vi "Register for Camera Events.vi"(8 "error in (no error)":errorcluster, 11 "Camera Controller in":refnum<class "Camera Controller.lvclass">) -> (0 "error out":errorcluster, 2 "output cluster":T1, 3 "Camera Controller out":refnum<class "Camera Controller.lvclass">)   [LabVIEW 2022 SP3, in "Camera Controller.lvclass"]
uses:
  Camera Controller.lvclass
  Camera Controller.lvclass/Camera Controller.ctl
  XY Stage/Process Actor/Process Framework/Process State Data/Process State Data.lvclass
  Camera Data/Camera Data.lvclass
  XY Stage/Process Actor/Process Framework/Process State Data/Events.ctl
  <vilib>/vision/Image Controls.llb/IMAQ Image.ctl
  Camera Data/events.ctl
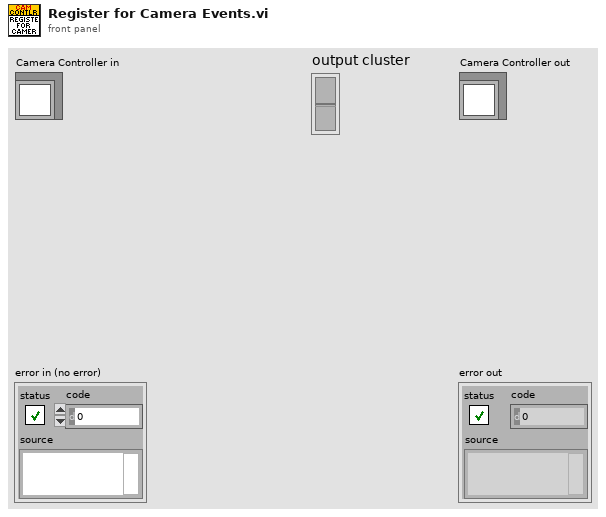
[diagram p1: front panel]
types:
  T1 = cluster{"Event Registration Refnum":refnum<event-registration>, "Event Registration Refnum":refnum<event-registration>}
  T2 = typedef "Camera Data.lvclass/events.ctl" = cluster{"Image":refnum<user-event>}
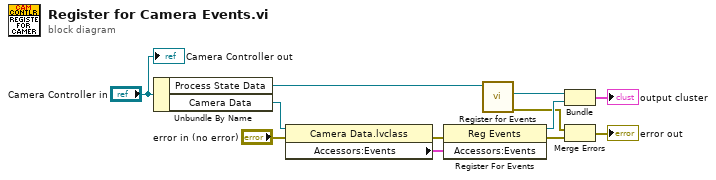
[diagram p0: block diagram]
diagram:
  n1 = Unbundle By Name("Camera Controller in") -> ("Process State Data"=w10:refnum<data-value>, "Camera Data"=w11:refnum<data-value>)
  n2 = property class="Camera Data.lvclass"(reference=w11, error in="error in (no error)") -> (error out=w4:errorcluster, "Accessors:Events"=w9:T2)  [unwired: 1 out]
  n3 = register-events(error in=w4, w9) -> (reference out=w8:refnum<event-registration>, error out=w2:errorcluster)  [unwired: 1 in]
  n4 = call "Register for Events.vi"("Process State"=w10) -> ("error out"=w3:errorcluster, "Event Registration Refnum"=w7:refnum<event-registration>)  [unwired: 8 in, 1 out]
  n5 = Bundle("Event Registration Refnum"=w7, "Event Registration Refnum"=w8) -> (→"output cluster":T1)  [unwired: 1 in]
  n6 = Merge Errors(w3, w2) -> (→"error out":errorcluster)
  "Camera Controller out" <- "Camera Controller in"
